vi "EOL CAN_Get Bootloader Key.vi"(7 "Rx Arbitration Id":u32=402522244 format="%.0x", 8 "Error in":errorcluster, 9 "SA2 Operator":T1[](array[typedef]) {"Wert" format="%.0x"}, 10 "Read Session in":refnum<k21>, 11 "Write Session in":refnum<k21>) -> (0 "Error out":errorcluster, 2 "Response Good?":bool, 3 "TxRx Data":string[][](array[string]))   [LabVIEW 2018]
uses:
  Typedefs/Diagnose_SA2_Rechnenbefehl.ctl
  Typedefs/Diagnose_SA2_Operation_ENUM.ctl
  <vilib>/xnet/xnet.llb/XNET Frame CAN.ctl
  <vilib>/xnet/xnet.llb/XNET Frame Type CAN.ctl
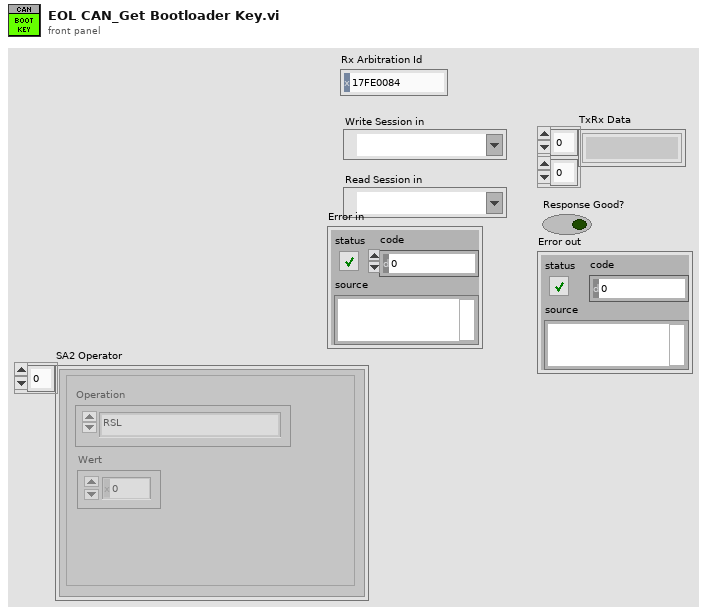
[diagram p1: front panel]
types:
  T1 = typedef "Diagnose_SA2_Rechnenbefehl.ctl" = cluster{"Operation":T2, "Wert":u32}
  T2 = typedef "Diagnose_SA2_Operation_ENUM.ctl" = enum16{"RSL", "RSR", "ADD", "SUB", "EOR", "Durchläufe", "NEXT", "BCC", "BRA", "Fertig"}
  T3 = typedef "XNET Frame CAN.ctl" = cluster{"timestamp":timestamp, "payload":u8[], "identifier":u32, "type":T4, "extended?":bool, "echo?":bool}
  T4 = typedef "XNET Frame Type CAN.ctl" = u8
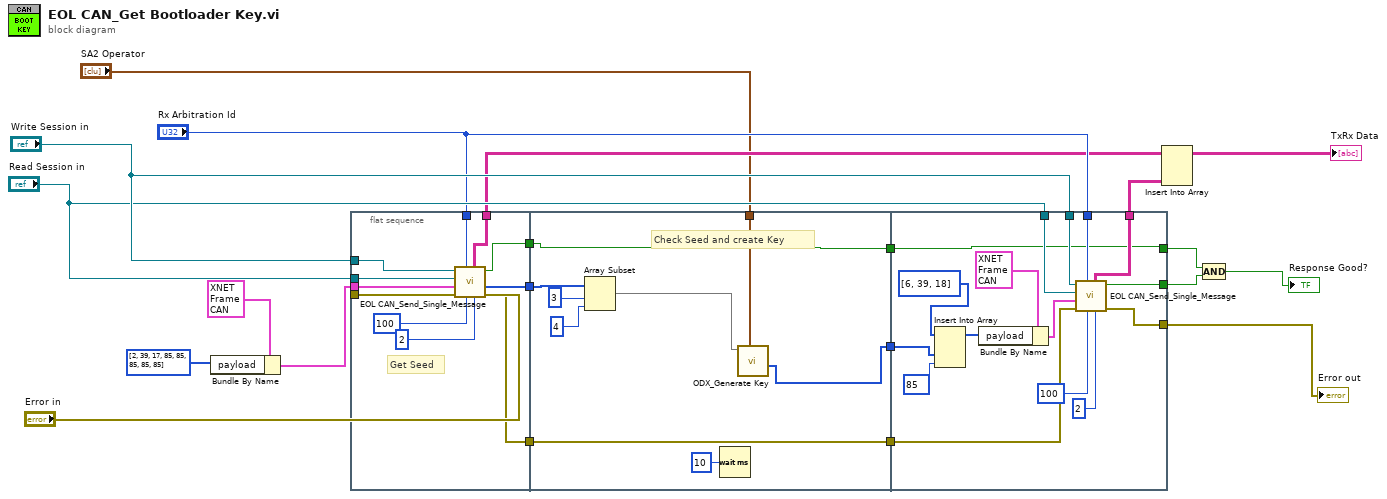
[diagram p0: block diagram]
diagram:
  n1 = Bundle By Name(cluster=T3 {"timestamp"=timestamp(0 s since 1904-01-01), "payload"=[2, 39, 3, 85, 85, 85, 85, 85], "identifier"=402391172, "type"=8, "extended?"=TRUE, "echo?"=FALSE} ("Tx CAN frame"), "payload"=u8[] [2, 39, 17, 85, 85, 85, 85, 85] ("Transmit Data 2")) -> (w19:T3)
  n2 = flat-sequence {
    tunnel: [w31] -> w9
    tunnel: w19 -> [w30]
    tunnel: "Read Session in" -> [w29]
    tunnel: "Write Session in" -> [w28]
    tunnel: "Error in" -> [w27]
    tunnel: "Rx Arbitration Id" -> [w25]
    tunnel: [w32] -> w17
    tunnel: [w26] -> w16
    tunnel: [w24] -> w14
    tunnel: w17 -> [w37]
    tunnel: w16 -> [w41]
    tunnel: [w41] -> w15
    tunnel: w14 -> [w40]
    tunnel: [w33] -> w13
    tunnel: [w37] -> w6
    tunnel: "SA2 Operator" -> [w34]
    tunnel: w15 -> [w57]
    tunnel: w13 -> [w49]
    tunnel: "Write Session in" -> [w54]
    tunnel: "Read Session in" -> [w53]
    tunnel: "Rx Arbitration Id" -> [w52]
    tunnel: [w51] -> w8
    tunnel: [w46] -> w3
    tunnel: w6 -> [w45]
    tunnel: [w45] -> w4
    tunnel: [w44] -> w2
    frame #0 {
      # "Get Seed"
      n3 = call "EOL CAN_Send_Single_Message.vi"("Retries"=2, "Msg Wait Time"=u32 100, "Rx Arbitration Id"=w25, "Error in"=w27, "Tx CAN frame"=w30, "Read Session in"=w29, "Write Session in"=w28) -> ("Error out"=w26:errorcluster, "Rx Message"=w24:u8[], "Response Good?"=w32:bool, "TxRx Data"=w31:string[][])  [unwired: 1 out]
    }
    frame #1 {
      # "Check Seed and create Key"
      n4 = Array Subset(array=w40, index=3, length=4) -> (w35:u8[])
      n5 = Wait (ms)(milliseconds to wait=u32 10) -> ()  [unwired: 1 out]
      n6 = call "ODX_Generate Key.vi"("SA2 Operator"=w34, "Responce with Seed"=w35) -> ("Key"=w33:u8[])  [unwired: 9 in]
    }
    frame #2 {
      n7 = Insert Into Array(array=u8[] [6, 39, 18] ("payload"), new element #1=w49, new element #2=u8 85 ("new element/subarray")) -> (w47:u8[])  [unwired: 1 in]
      n8 = Bundle By Name(cluster=T3 {"timestamp"=timestamp(0 s since 1904-01-01), "payload"=[2, 39, 3, 85, 85, 85, 85, 85], "identifier"=402391172, "type"=8, "extended?"=TRUE, "echo?"=FALSE} ("Tx CAN frame"), "payload"=w47) -> (w55:T3)
      n9 = call "EOL CAN_Send_Single_Message.vi"("Retries"=2, "Msg Wait Time"=u32 100, "Rx Arbitration Id"=w52, "Error in"=w57, "Tx CAN frame"=w55, "Read Session in"=w53, "Write Session in"=w54) -> ("Error out"=w44:errorcluster, "Response Good?"=w46:bool, "TxRx Data"=w51:string[][])  [unwired: 2 out]
    }
  }
  n10 = Insert Into Array(array=w9, new element=w8) -> (→"TxRx Data":string[][])  [unwired: 2 in]
  n11 = Compound Arithmetic op=AND(w4, w3) -> (→"Response Good?":bool)
  "Error out" <- w2
